vi "Query Multi Eval Meas List ES Flatness Limit Check Results.vi"(6 "Difference (Difference 1)":T1=1 items=["Difference 1"=1, "Difference 2"=2], 8 "error in (no error)":errorcluster, 9 "Result Type (Current)":i32(ring) items=["Current", "Average", "Extreme"], 10 "Instance (1)":T2=1, 11 "VISA resource name":refnum<visa-resource-name>) -> (0 "error out":errorcluster, 1 "Limit Check Results":i32[](array[numeric]), 2 "Reliability":i32, 3 "VISA resource name out":refnum<visa-resource-name>)   [LabVIEW 2020, in "Rohde&Schwarz CMWXP NR FR1 Measurement.lvlib"]
doc: "Return equalizer spectrum flatness single value limit check results (differences between ranges) for all measured list mode segments.\n\nAttributes:\nRSCMWXPNRFR1M_ATTR_QUERY_MULTI_EVAL_MEAS_LIST_ES_FLATNESS_CURRENT_LIMIT_CHECK_RESULTS\nRSCMWXPNRFR1M_ATTR_QUERY_MULTI_EVAL_MEAS_LIST_ES_FLATNESS_AVERAGE_LIMIT_CHECK_RESULTS\nRSCMWXPNRFR1M_ATTR_QUERY_MULTI_EVAL_MEAS_LIST_ES_FLATNESS_EXTREME_LIMIT_CHECK_RESULTS\n\nRemote-control commands:\nCALCulate:NRSub:MEAS<i>:MEValuation:LIST:ESFLatness:DIFFerence<no>:CURRent?\nCALCulate:NRSub:MEAS<i>:MEValuation:LIST:ESFLatness:DIFFerence<no>:AVERage?\nCALCulate:NRSub:MEAS<i>:MEValuation:LIST:ESFLatness:DIFFerence<no>:EXTReme?"
uses:
  <instrlib>/Rohde&Schwarz CMWXP NR FR1 Measurement/Rohde&Schwarz CMWXP NR FR1 Measurement.lvlib
  <instrlib>/Rohde&Schwarz CMWXP NR FR1 Measurement/Private/_Instance.ctl
  <instrlib>/Rohde&Schwarz CMWXP NR FR1 Measurement/Private/_Difference.ctl
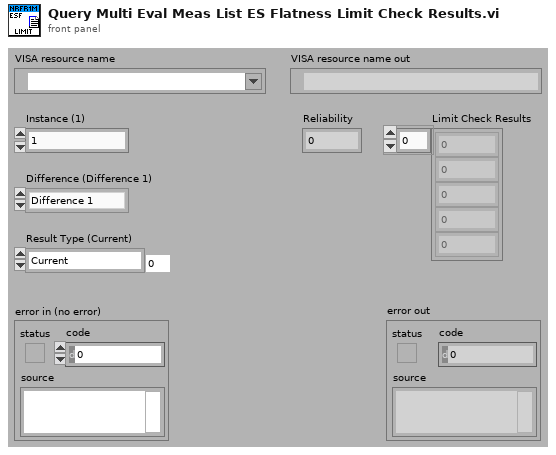
[diagram p1: front panel]
types:
  T1 = typedef "Rohde&Schwarz CMWXP NR FR1 Measurement.lvlib/_Difference.ctl" = i32
  T2 = typedef "Rohde&Schwarz CMWXP NR FR1 Measurement.lvlib/_Instance.ctl" = i32
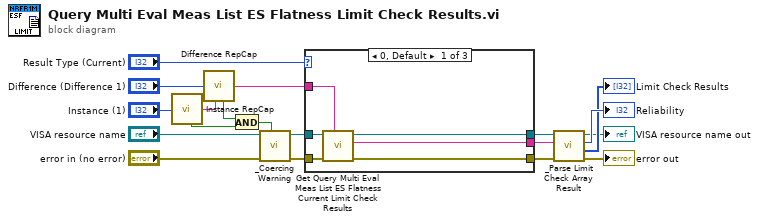
[diagram p0: block diagram]
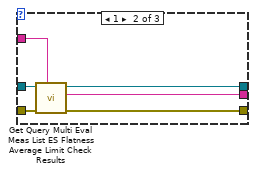
[diagram p2: hidden frame]
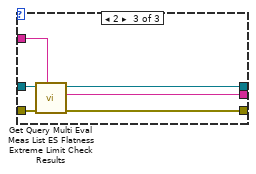
[diagram p3: hidden frame]
diagram:
  n1 = call <instrlib>:"Instance RepCap.vi"("Instance In"="Instance (1)") -> ("In Range?"=w14:bool, "RepCap Identifier Out"=w15:string)  [unwired: 1 in]
  n2 = call <instrlib>:"Difference RepCap.vi"("Difference In"="Difference (Difference 1)", "RepCap String In (\"\")"=w15) -> ("In Range?"=w13:bool, "RepCap Identifier Out"=w10:string)
  n3 = And(x=w13, y=w14) -> (x .and. y?=w17:bool)
  n4 = call <instrlib>:"_Coercing Warning.vi"("In Range?"=w17, "error in (no error)"="error in (no error)", "VISA resource name"="VISA resource name") -> ("error out"=w11:errorcluster, "VISA resource name out"=w12:refnum<visa-resource-name>)  [unwired: 7 in]
  n5 = case shown="0, Default" "Result Type (Current)" {
    tunnel: w12 -> [w25 w31 w37]
    tunnel: w11 -> [w24 w30 w36]
    tunnel: w10 -> [w23 w29 w35]
    tunnel: [w22 w28 w34] -> w6
    tunnel: [w21 w27 w33] -> w7
    tunnel: [w20 w26 w32] -> w8
    frame 0, Default {
      n6 = call "Get Query Multi Eval Meas List ES Flatness Current Limit Check Results"("Repeated Capabilities"=w23, "error in (no error)"=w24, "instrument handle"=w25) -> ("error out"=w20:errorcluster, "Query Multi Eval Meas List ES Flatness Current Limit Check Results"=w21:string, "instrument handle out"=w22:refnum<visa-resource-name>)  [unwired: 6 in]
    }
    frame 1 {
      n7 = call "Get Query Multi Eval Meas List ES Flatness Average Limit Check Results"("Repeated Capabilities"=w29, "error in (no error)"=w30, "instrument handle"=w31) -> ("error out"=w26:errorcluster, "Query Multi Eval Meas List ES Flatness Average Limit Check Results"=w27:string, "instrument handle out"=w28:refnum<visa-resource-name>)  [unwired: 6 in]
    }
    frame 2 {
      n8 = call "Get Query Multi Eval Meas List ES Flatness Extreme Limit Check Results"("Repeated Capabilities"=w35, "error in (no error)"=w36, "instrument handle"=w37) -> ("error out"=w32:errorcluster, "Query Multi Eval Meas List ES Flatness Extreme Limit Check Results"=w33:string, "instrument handle out"=w34:refnum<visa-resource-name>)  [unwired: 6 in]
    }
  }
  n9 = call <instrlib>:"_Parse Limit Check Array Result.vi"("error in (no error)"=w8, "Input String"=w7, "VISA resource name"=w6) -> ("error out"=→"error out":errorcluster, "Results"=→"Limit Check Results":i32[], "Reliability"=→"Reliability":i32, "VISA resource name out"=→"VISA resource name out":refnum<visa-resource-name>)  [unwired: 3 in, 1 out]
